vi "Create.vi"(10 "Load Result":T1) -> (3 "Load Result Value out":refnum<class "Load Result Value.lvclass">)   [LabVIEW 2020, in "VolatusSeq.lvlib" / "Load Result Value.lvclass"]
uses:
  Load Result Value.lvclass
  Load Result.ctl
  Load Result Value.lvclass/Load Result Value.ctl
  VolatusSeq.lvlib
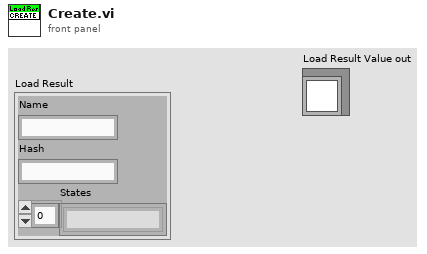
[diagram p1: front panel]
types:
  T1 = typedef "VolatusSeq.lvlib/Load Result.ctl" = cluster{"Name":string, "Hash":string, "States":string[]}
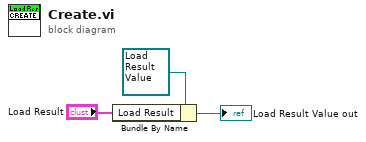
[diagram p0: block diagram]
diagram:
  n1 = Bundle By Name(cluster=refnum<class "Load Result Value.lvclass"> refnum ("Load Result Value in"), "Load Result"="Load Result") -> (→"Load Result Value out":refnum<class "Load Result Value.lvclass">)
